vi "PenaltyDefenseSkill.vi"(4 "Game in":refnum<class "Game.lvclass">, 6 "PenaltyOurKick?":bool, 8 "error in (no error)":errorcluster, 9 "IndexInVector":dbl, 10 "Robot":refnum<class "Robot.lvclass">, 11 "PenaltyDefenseSkill in":refnum<class "PenaltyDefenseSkill.lvclass">) -> (0 "error out":errorcluster, 2 "Robot out":refnum<class "Robot.lvclass">, 3 "PenaltyDefenseSkill out":refnum<class "PenaltyDefenseSkill.lvclass">)   [LabVIEW 2020, in "PenaltyDefenseSkill.lvclass"]
uses:
  PenaltyDefenseSkill.lvclass
  Robot_class/Robot.lvclass
  C:/RoboIME/SSL_AI/Object_class/Object.lvclass
  Game_class/Game.lvclass
  Game_class/Game.lvclass/Game.ctl
  Team_class/Team.lvclass/Team.ctl
  Object_class/Object.lvclass/Object.ctl
  Robot_class/Robot.lvclass/Robot.ctl
  Object_class/Read position(x,y).vi
  Game_class/Read FieldRef.vi
  Game_class/Read NewParameters.vi
  Game_class/Read EnemyRef.vi
  Game_class/Read AllyRef.vi
  Game_class/Read Referee.vi
  Referee_class/Read our_goalie_id.vi
  Referee_class/Read enemy_goalie_id.vi
  Team_class/Read RobotRef.vi
  Robot_class/Write dest_x.vi
  Robot_class/Write dest_y.vi
  Robot_class/Write dest_orientation.vi
  Ally_class/Ally.lvclass
  C:/RoboIME/SSL_AI/Team_class/Team.lvclass
  Enemy_class/Enemy.lvclass
  Field_class/Field.lvclass
  Referee_class/Referee.lvclass
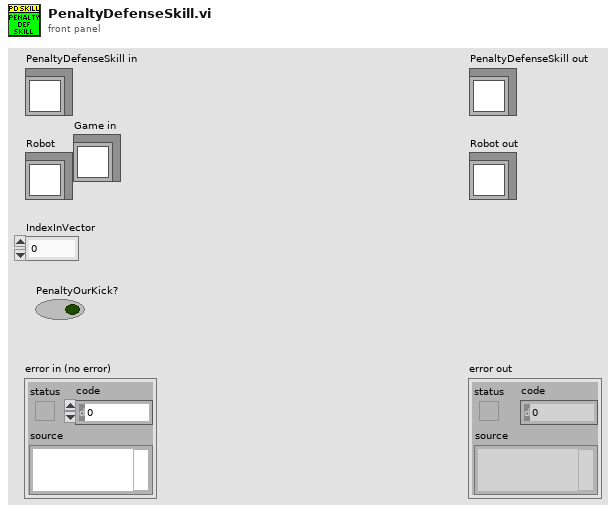
[diagram p1: front panel]
types:
  T1 = typedef "NewParameters.ctl" = cluster{"PenaltyDistance":dbl, "DistanceAttackerToBackBall":dbl, "Division":enum16{"Div B", "Div A"}, "DistanceToAvoidyEnemyRobot":dbl, "BallPlacementDistance":dbl, "DisatanceBehindBallToStealBall":dbl}
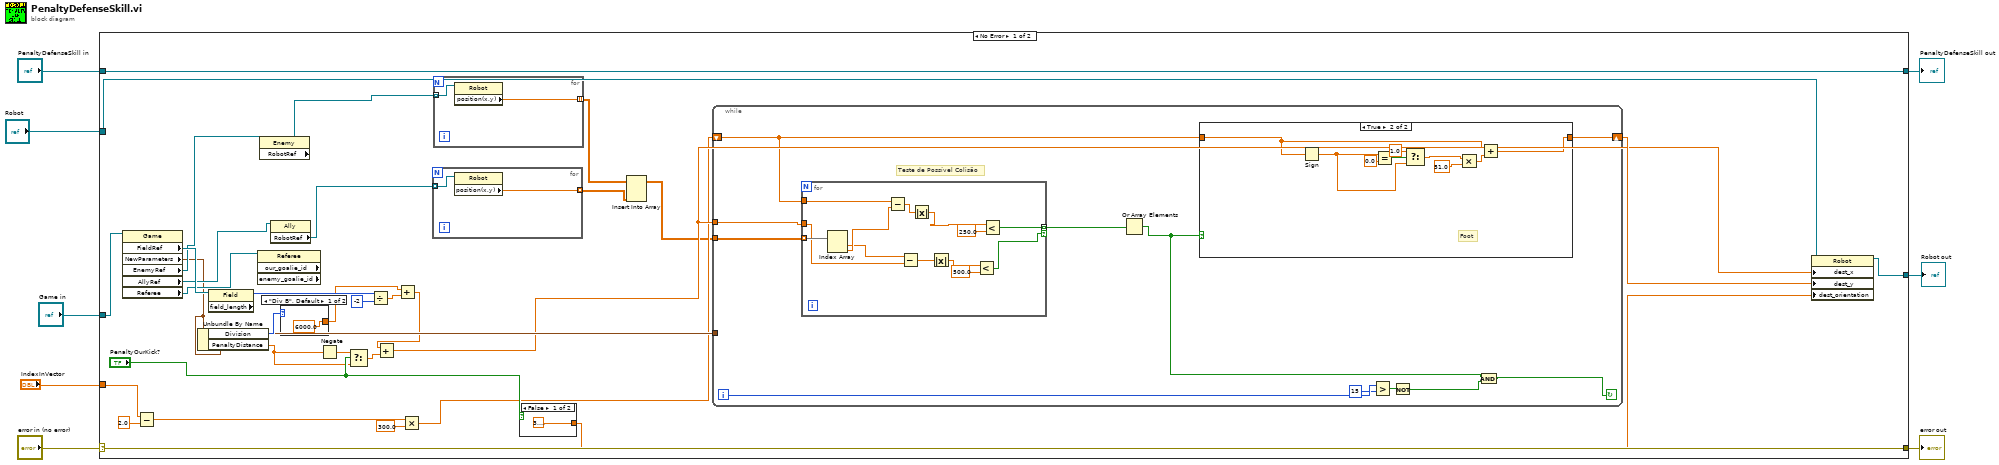
[diagram p0: block diagram]
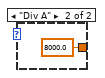
[diagram p2: hidden frame]
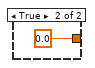
[diagram p3: hidden frame]
diagram:
  n1 = case shown="No Error" "error in (no error)" {
    selector: "error in (no error)" -> [w40 w86]
    tunnel: [w40 w86] -> w7
    tunnel: [w41 w85] -> w5
    tunnel: "PenaltyDefenseSkill in" -> [w41 w85]
    tunnel: "IndexInVector" -> [w13 _]
    tunnel: "Robot" -> [w17 w84]
    tunnel: [w39 w84] -> w2
    tunnel: "Game in" -> [w38 _]
    frame No Error {
      n2 = property class="Game"(reference=w38) -> ("FieldRef"=w33:refnum<class "Field.lvclass">, "NewParameters"=w21:T1, "EnemyRef"=w27:refnum<class "Enemy.lvclass">, "AllyRef"=w26:refnum<class "Ally.lvclass">, "Referee"=w24:refnum<class "Referee.lvclass">)  [unwired: 1 in, 2 out]
      n3 = Subtract(x=w13, y=2.0) -> (x-y=w12:dbl)
      n4 = Unbundle By Name(w21) -> ("Division"=w29:enum16{"Div B", "Div A"}, "PenaltyDistance"=w34:dbl)
      n5 = property class="Field"(reference=w33) -> ("field_length"=w32:i32)  [unwired: 1 in, 2 out]
      n6 = property class="Referee" props=["our_goalie_id", "enemy_goalie_id"](reference=w24) -> ()  [unwired: 1 in, 4 out]
      n7 = property class="Enemy"(reference=w27) -> ("RobotRef"=w25:refnum<class "Robot.lvclass">[])  [unwired: 1 in, 2 out]
      n8 = property class="Ally"(reference=w26) -> ("RobotRef"=w23:refnum<class "Robot.lvclass">[])  [unwired: 1 in, 2 out]
      n9 = case shown="\"Div B\", Default" w29 {
        tunnel: [6000.0 8000.0] -> w28
        frame "Div B", Default {
        }
        frame "Div A" {
        }
      }
      n10 = Negate(x=w34) -> (-x=w36:dbl)
      n11 = Select(t=w36, s="PenaltyOurKick?", f=w34) -> (s? t:f=w35:dbl)
      n12 = Divide(x=w32, y=-2) -> (x/y=w30:dbl)
      n13 = Add(x=w28, y=w30) -> (x+y=w20:dbl)
      n14 = Add(x=w20, y=w35) -> (x+y=w15:dbl)
      n15 = Multiply(x=w12, y=300.0) -> (x*y=w10:dbl)
      n16 = for {
        tunnel: w23 -> [w43] mode=indexing
        tunnel: [w42] -> w22 mode=indexing
        n17 = property class="Robot"(reference=w43) -> ("position(x,y)"=w42:dbl[])  [unwired: 1 in, 2 out]
      }
      n18 = for {
        tunnel: w25 -> [w45] mode=indexing
        tunnel: [w44] -> w16 mode=indexing
        n19 = property class="Robot"(reference=w45) -> ("position(x,y)"=w44:dbl[])  [unwired: 1 in, 2 out]
      }
      n20 = case shown="False" "PenaltyOurKick?" {
        tunnel: [3.141592653589793 0.0 ("x")] -> w19
        frame False {
        }
        frame True {
        }
      }
      n21 = Insert Into Array(array=w16, new element=w22) -> (w9:dbl[][])  [unwired: 2 in]
      n22 = while {
        shift-right: [w53] -> w18
        shift-left: w10 -> [w52]
        tunnel: w9 -> [w51]
        tunnel: w21 -> [_]
        tunnel: w15 -> [w50]
        i -> [w58]
        stop <- w56 continue-if-true
        # "Teste de Possível Colisão"
        n23 = for {
          tunnel: [w73] -> w60 mode=indexing if=w65
          tunnel: w51 -> [w71] mode=indexing
          tunnel: w52 -> [w72]
          tunnel: w50 -> [w68]
          n24 = Index Array(array=w71) -> (element #1=w69:dbl, element #2=w70:dbl)  [unwired: 2 in]
          n25 = Subtract(x=w72, y=w70) -> (x-y=w62:dbl)
          n26 = Subtract(x=w69, y=w68) -> (x-y=w67:dbl)
          n27 = Absolute Value(x=w62) -> (abs(x)=w61:dbl)
          n28 = Absolute Value(x=w67) -> (abs(x)=w66:dbl)
          n29 = Less?(x=w66, y=500.0) -> (x < y?=w65:bool)
          n30 = Less?(x=w61, y=250.0) -> (x < y?=w73:bool)
        }
        n31 = Or Array Elements(Boolean array=w60) -> (logical OR=w55:bool)
        n32 = case shown="True" w55 {
          tunnel: w52 -> [w74 w77]
          tunnel: [w74 w83] -> w53
          frame False {
          }
          frame True {
            # "Foot"
            n33 = Sign(1:w77) -> (0:w75:dbl)
            n34 = Equal?(x=w75, y=0.0) -> (x = y?=w79:bool)
            n35 = Select(t=1.0, s=w79, f=w75) -> (s? t:f=w76:dbl)
            n36 = Multiply(x=w76, y=51.0 ("element")) -> (x*y=w82:dbl)
            n37 = Add(x=w77, y=w82) -> (x+y=w83:dbl)
          }
        }
        n38 = Greater?(x=w58, y=15) -> (0:w59:bool)
        n39 = Not(x=w59) -> (.not. x?=w54:bool)
        n40 = And(x=w55, y=w54) -> (x .and. y?=w56:bool)
      }
      n41 = property class="Robot"(reference=w17, "dest_x"=w15, "dest_y"=w18, "dest_orientation"=w19) -> (reference out=w39:refnum<class "Robot.lvclass">)  [unwired: 1 in, 1 out]
    }
    frame Error {
    }
  }
  "error out" <- w7
  "PenaltyDefenseSkill out" <- w5
  "Robot out" <- w2
